vi "synnax client close.vi"(8 "error in":errorcluster, 11 "client":u64) -> (0 "error out":errorcluster)   [LabVIEW 2026, in "synnax_lib.lvlib" / "Synnax Client.lvclass"]
doc: "SYNNAX_EXPORT void synnax_client_close(SynnaxClient client);"
uses:
  Synnax Client.lvclass
  Synnax Client.lvclass/Synnax Client.ctl
  synnax_clib.dll
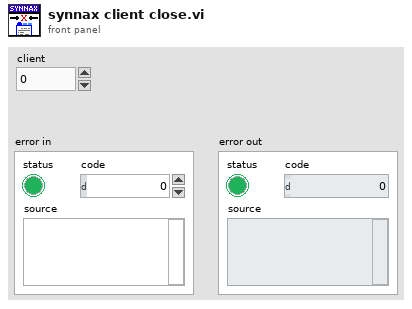
[diagram p1: front panel]
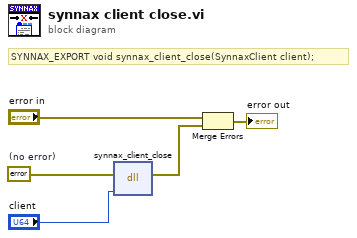
[diagram p0: block diagram]
diagram:
  w1 = errorcluster {"status"=FALSE, "code"=0, "source"=""}  # (no error)
  # "SYNNAX_EXPORT void synnax_client_close(SynnaxClient client);"
  n1 = dll-call lib="C/synnax/client/lv/synnax_clib.*" fn="synnax_client_close"(error in=w1, "client"="client") -> (error out=w4:errorcluster)  [unwired: 4 in, 1 out]
  n2 = Merge Errors("error in", w4) -> (→"error out":errorcluster)
